vi "GenerationConfig.vi"(8 "error in (no error)":errorcluster, 11 "GenerationConfig":T3={"ExternalAtt"=0.0, "Freq"=5180000000.0, "RxPwr"=-40.0, "PacketNumber"=100, "WaveformName(WithType)"="ac80mcs9.tdms", "PhyPort"=enum."Port5", "PhyPort2"=enum."Port5", "Freq2"=5180000000.0, "BW"=enum."5M", "MCSIndex"=7.0} {"Freq2" format="%#_13g"; "RxPwr" format="%#_13g"; "Freq" format="%#_13g"; "ExternalAtt" format="%#_13g"}) -> (0 "error out":errorcluster, 3 "GenerationConfigCMD":string[](array[string])=["SOUR:RFSG:GPRF:EATTenuation 0", "SOUR:RFSG:GPRF:FREQ 5180000000", "SOUR:RFSG:GPRF:LEVel -40", "SOUR:RFSG:GPRF:PORT 'Port5'", "SOUR:RFSG:GPRF:ARB:CYCL 100", "SOUR:RFSG:GPRF:ARB:REP FINITE", "SOUR:RFSG:GPRF:ARB:WAV 'ac80mcs9.tdms'", "SOUR:RFSG:GPRF:MODE  ARB", "*OPC?"])   [LabVIEW 2015]
uses:
  PhyPort.ctl
  BW.ctl
panel:
  out "size(s)":i32
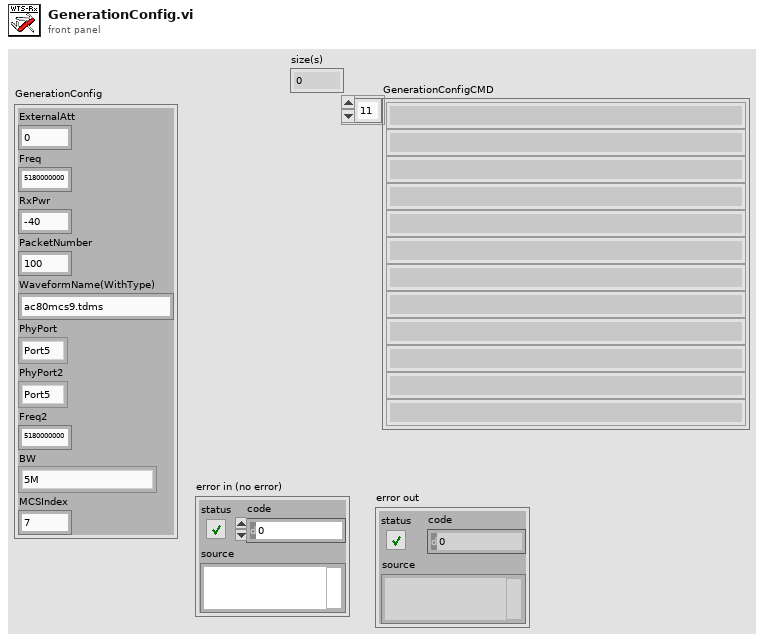
[diagram p1: front panel]
types:
  T1 = typedef "PhyPort.ctl" = enum16{"Port0", "Port1", "Port2", "Port3", "Port4", "Port5", "Port6", "Port7"}
  T2 = typedef "BW.ctl" = enum16{"5M", "10M", "20M", "40M", "80M", "80P80M", "160M"}
  T3 = cluster{"ExternalAtt":dbl, "Freq":dbl, "RxPwr":dbl, "PacketNumber":i32, "WaveformName(WithType)":string, "PhyPort":T1, "PhyPort2":T1, "Freq2":dbl, "BW":T2, "MCSIndex":dbl}
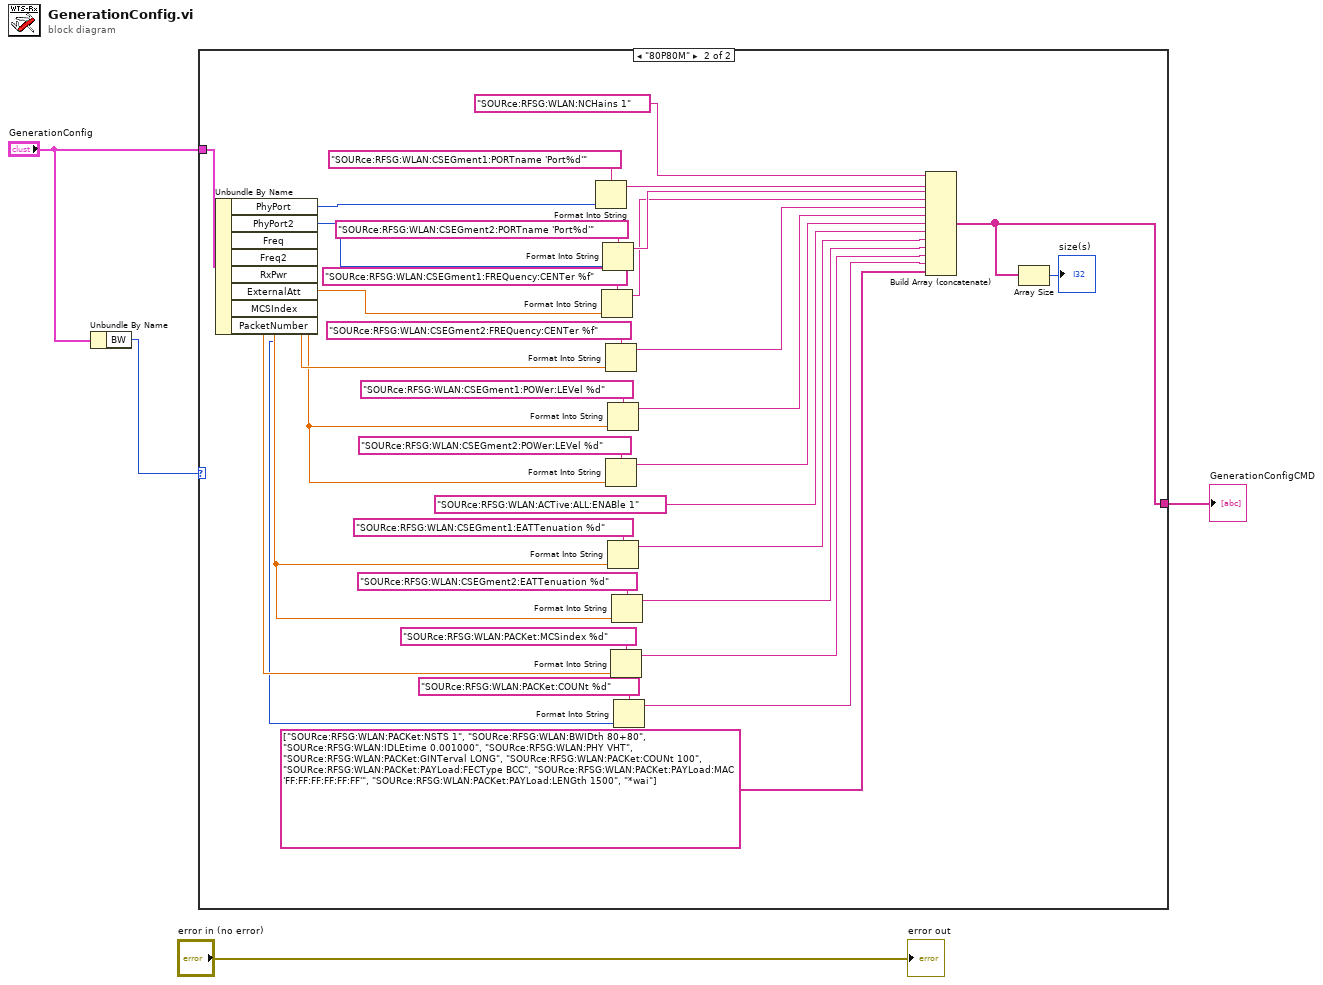
[diagram p0: block diagram]
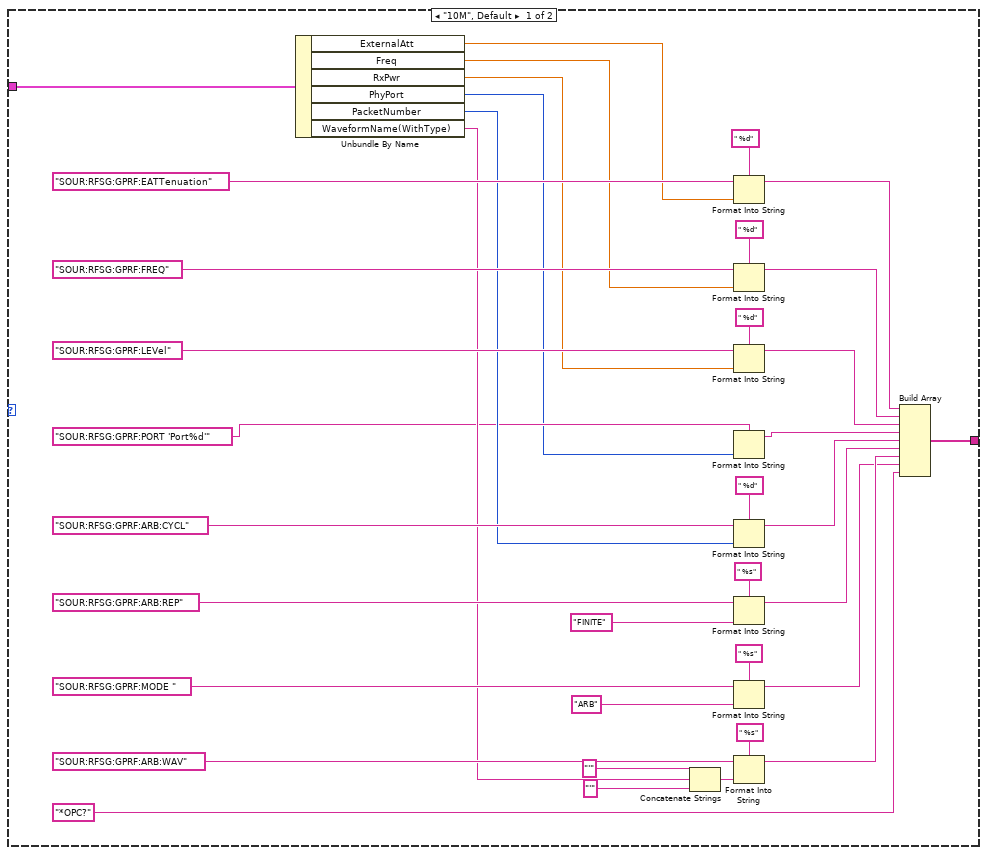
[diagram p2: hidden frame]
diagram:
  n1 = Unbundle By Name("GenerationConfig") -> ("BW"=w1:T2)
  n2 = case shown="\"80P80M\"" w1 {
    tunnel: [w13 w43] -> w4
    tunnel: "GenerationConfig" -> [w12 w74]
    frame "10M", Default {
      n3 = Unbundle By Name(w12) -> ("ExternalAtt"=w11:dbl, "Freq"=w10:dbl, "RxPwr"=w9:dbl, "PhyPort"=w5:T1, "PacketNumber"=w8:i32, "WaveformName(WithType)"=w7:string)
      n4 = Concatenate Strings("'", w7, "'" ("string")) -> (w25:string)
      n5 = Format Into String(format string=" %d", initial string="SOUR:RFSG:GPRF:EATTenuation", w11) -> (resulting string=w24:string)  [unwired: 1 in, 1 out]
      n6 = Format Into String(format string=" %d", initial string="SOUR:RFSG:GPRF:FREQ", w10) -> (resulting string=w23:string)  [unwired: 1 in, 1 out]
      n7 = Format Into String(format string=" %d", initial string="SOUR:RFSG:GPRF:LEVel", w9) -> (resulting string=w22:string)  [unwired: 1 in, 1 out]
      n8 = Format Into String(format string="SOUR:RFSG:GPRF:PORT 'Port%d'" ("initial string"), w5) -> (resulting string=w21:string)  [unwired: 2 in, 1 out]
      n9 = Format Into String(format string=" %d", initial string="SOUR:RFSG:GPRF:ARB:CYCL", w8) -> (resulting string=w20:string)  [unwired: 1 in, 1 out]
      n10 = Format Into String(format string=" %s", initial string="SOUR:RFSG:GPRF:ARB:REP", "FINITE" ("input 1")) -> (resulting string=w19:string)  [unwired: 1 in, 1 out]
      n11 = Format Into String(format string=" %s", initial string="SOUR:RFSG:GPRF:MODE ", "ARB" ("input 1")) -> (resulting string=w17:string)  [unwired: 1 in, 1 out]
      n12 = Format Into String(format string=" %s", initial string="SOUR:RFSG:GPRF:ARB:WAV", w25) -> (resulting string=w18:string)  [unwired: 1 in, 1 out]
      n13 = Build Array(w24, w23, w22, w21, w20, w19, w18, w17, "*OPC?") -> (w13:string[])
    }
    frame "80P80M" {
      n14 = Unbundle By Name(w74) -> ("PhyPort"=w72:T1, "PhyPort2"=w71:T1, "Freq"=w69:dbl, "Freq2"=w67:dbl, "RxPwr"=w60:dbl, "ExternalAtt"=w52:dbl, "MCSIndex"=w49:dbl, "PacketNumber"=w46:i32)
      n15 = Format Into String(format string="SOURce:RFSG:WLAN:CSEGment1:PORTname 'Port%d'", w72) -> (resulting string=w66:string)  [unwired: 2 in, 1 out]
      n16 = Format Into String(format string="SOURce:RFSG:WLAN:CSEGment1:FREQuency:CENTer %f", w69) -> (resulting string=w64:string)  [unwired: 2 in, 1 out]
      n17 = Format Into String(format string="SOURce:RFSG:WLAN:CSEGment2:PORTname 'Port%d'", w71) -> (resulting string=w65:string)  [unwired: 2 in, 1 out]
      n18 = Format Into String(format string="SOURce:RFSG:WLAN:CSEGment2:FREQuency:CENTer %f", w67) -> (resulting string=w63:string)  [unwired: 2 in, 1 out]
      n19 = Format Into String(format string="SOURce:RFSG:WLAN:CSEGment2:POWer:LEVel %d", w60) -> (resulting string=w58:string)  [unwired: 2 in, 1 out]
      n20 = Format Into String(format string="SOURce:RFSG:WLAN:CSEGment1:POWer:LEVel %d", w60) -> (resulting string=w59:string)  [unwired: 2 in, 1 out]
      n21 = Format Into String(format string="SOURce:RFSG:WLAN:CSEGment1:EATTenuation %d", w52) -> (resulting string=w54:string)  [unwired: 2 in, 1 out]
      n22 = Format Into String(format string="SOURce:RFSG:WLAN:PACKet:MCSindex %d", w49) -> (resulting string=w48:string)  [unwired: 2 in, 1 out]
      n23 = Format Into String(format string="SOURce:RFSG:WLAN:CSEGment2:EATTenuation %d", w52) -> (resulting string=w51:string)  [unwired: 2 in, 1 out]
      n24 = Format Into String(format string="SOURce:RFSG:WLAN:PACKet:COUNt %d", w46) -> (resulting string=w45:string)  [unwired: 2 in, 1 out]
      n25 = Build Array (concatenate)("SOURce:RFSG:WLAN:NCHains 1", w66, w65, w64, w63, w59, w58, "SOURce:RFSG:WLAN:ACTive:ALL:ENABle 1", w54, w51, w48, w45, string[] ["SOURce:RFSG:WLAN:PACKet:NSTS 1", "SOURce:RFSG:WLAN:BWIDth 80+80", "SOURce:RFSG:WLAN:IDLEtime 0.001000", "SOURce:RFSG:WLAN:PHY VHT", "SOURce:RFSG:WLAN:PACKet:GINTerval LONG", "SOURce:RFSG:WLAN:PACKet:COUNt 100", "SOURce:RFSG:WLAN:PACKet:PAYLoad:FECType BCC", "SOURce:RFSG:WLAN:PACKet:PAYLoad:MAC 'FF:FF:FF:FF:FF:FF'", "SOURce:RFSG:WLAN:PACKet:PAYLoad:LENGth 1500", "*wai"]) -> (w43:string[])
      n26 = Array Size(array=w43) -> (size(s)=→"size(s)":i32)
    }
  }
  "GenerationConfigCMD" <- w4
  "error out" <- "error in (no error)"
